vi "Manual Triggered Apodization 2.vi"() -> ()   [LabVIEW 2012]
uses:
  LabVIEW/user.lib/SpectralRadar.llb/Processing Parameter Int Selection.ctl
  LabVIEW/user.lib/SpectralRadar.llb/Calibration Selection.ctl
  LabVIEW/user.lib/SpectralRadar.llb/set Spectrum Output.vi
  LabVIEW/user.lib/SpectralRadar.llb/display Data 1D.vi
  LabVIEW/user.lib/SpectralRadar.llb/OCT Device.lvclass
  LabVIEW/user.lib/SpectralRadar.llb/Processing.lvclass
  LabVIEW/user.lib/SpectralRadar.llb/Raw Data.lvclass
  LabVIEW/user.lib/SpectralRadar.llb/Data.lvclass
panel:
  out "Waveform Graph":dbl[](graph)
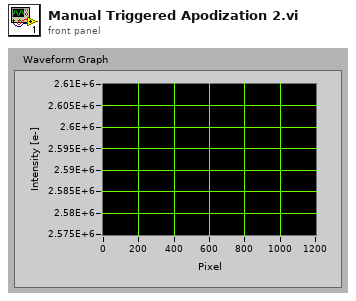
[diagram p1: front panel]
types:
  T1 = typedef "Processing.lvclass/Calibration Selection.ctl" = enum16{"Offset Errors", "Apodization Spectrum", "Apodization Vector", "Dispersion", "Chirp", "Extended Adjust", "Fixed Pattern"}
  T2 = typedef "Processing.lvclass/Processing Parameter Int Selection.ctl" = enum32{"Spectrum Averaging", "A-Scan Averaging", "B-Scan Averaging", "Zero Padding", "Number of Threads", "Fourier Averaging"}
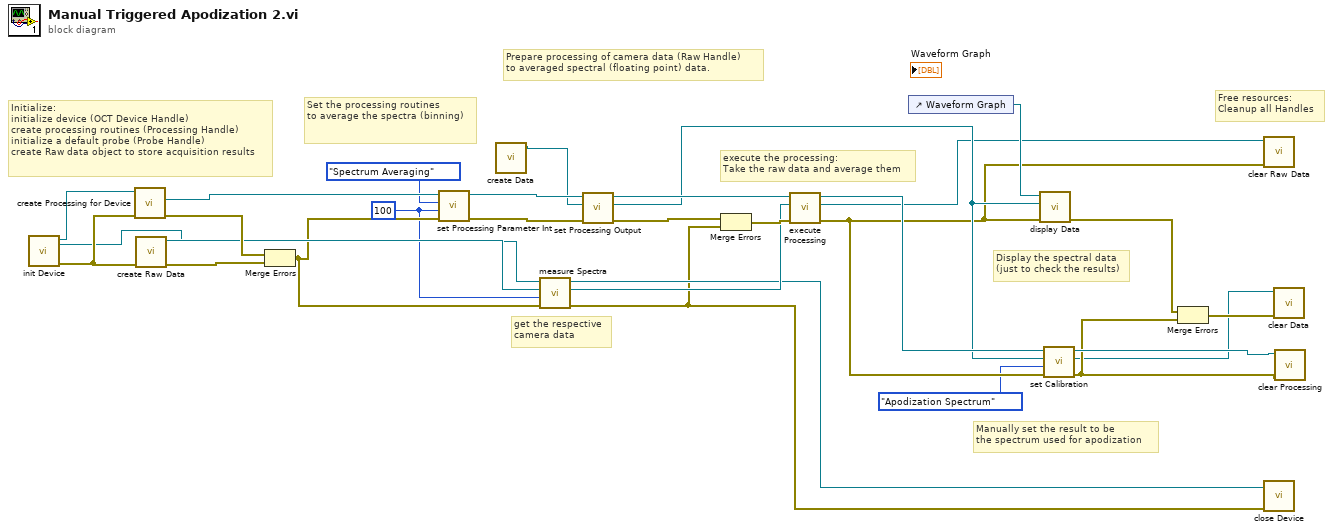
[diagram p0: block diagram]
diagram:
  w10 = 100 ("AScans")
  # "Free resources:\nCleanup all Handles"
  # "Manually set the result to be \nthe spectrum used for apodization"
  # "Display the spectral data\n(just to check the results)"
  # "execute the processing:\nTake the raw data and average them"
  # "get the respective \ncamera data"
  # "Prepare processing of camera data (Raw Handle)\nto averaged spectral (floating point) data."
  # "Set the processing routines \nto average the spectra (binning)"
  # "Initialize:\ninitialize device (OCT Device Handle)\ncreate processing routines (Processing Handle)\ninitialize a default probe (Probe Handle)\ncreate Raw data object to store acquisition results"
  n1 = call "init Device.vi"() -> ("error out"=w29:errorcluster, "OCTDevice"=w6:refnum<class "OCT Device.lvclass">)  [unwired: 6 in]
  n2 = call "create Processing for Device.vi"("error in (no error)"=w29, "OCTDevice"=w6) -> ("error out"=w27:errorcluster, "Processing"=w28:refnum<class "Processing.lvclass">)  [unwired: 3 in, 1 out]
  n3 = call "create Raw Data.vi"("error in (no error)"=w29) -> ("error out"=w26:errorcluster, "Raw Data"=w13:refnum<class "Raw Data.lvclass">)  [unwired: 5 in]
  n4 = Merge Errors(w27, w26) -> (w11:errorcluster)
  n5 = call "set Processing Parameter Int.vi"("error in (no error)"=w11, "Value"=w10, "Processing Paramter Int Selection"=Processing_Parameter_Int_Selection."Spectrum Averaging", "Processing in"=w28) -> ("error out"=w23:errorcluster, "Processing out"=w25:refnum<class "Processing.lvclass">)  [unwired: 2 in]
  n6 = call "create Data.vi"() -> ("Data"=w5:refnum<class "Data.lvclass">)  [unwired: 6 in, 1 out]
  n7 = call "measure Spectra.vi"("error in (no error)"=w11, "NumberOfSpectra"=w10, "Raw Data"=w13, "OCTDevice"=w6) -> ("error out"=w8:errorcluster, "Raw Data"=w12:refnum<class "Raw Data.lvclass">, "OCTDevice"=w9:refnum<class "OCT Device.lvclass">)  [unwired: 2 in]
  n8 = call-poly "set Processing Output.vi"("error in (no error)"=w23, "Data"=w5, "Processing"=w25) -> ("error out"=w15:errorcluster, "Data"=w19:refnum<class "Data.lvclass">, "Processing"=w22:refnum<class "Processing.lvclass">)  [unwired: 2 in]
  n9 = Merge Errors(w15, w8) -> (w14:errorcluster)
  n10 = call "execute Processing.vi"("error in (no error)"=w14, "Raw Data"=w12, "Processing"=w22) -> ("error out"=w16:errorcluster, "Raw Data"=w18:refnum<class "Raw Data.lvclass">, "Processing"=w20:refnum<class "Processing.lvclass">)  [unwired: 2 in]
  n11 = control-ref of="Waveform Graph"() -> (w21:refnum<vi>)
  n12 = call-poly "display Data.vi"("error in (no error)"=w16, "Data in"=w19, "WFGraph Refnum"=w21) -> ("error out"=w17:errorcluster)  [unwired: 2 in, 2 out]
  n13 = call "set Calibration.vi"("error in (no error)"=w16, "Calibration Data"=Calibration_Selection."Apodization Spectrum", "Data"=w19, "Processing"=w20) -> ("error out"=w3:errorcluster, "Data"=w1:refnum<class "Data.lvclass">, "Processing"=w4:refnum<class "Processing.lvclass">)  [unwired: 1 in]
  n14 = Merge Errors(w17, w3) -> (w2:errorcluster)
  n15 = call "clear Raw Data.vi"("error in (no error)"=w16, "Raw Data"=w18) -> ()  [unwired: 5 in, 1 out]
  n16 = call "close Device.vi"("error in (no error)"=w8, "OCTDevice"=w9) -> ()  [unwired: 5 in, 1 out]
  n17 = call "clear Data.vi"("error in (no error)"=w2, "Data"=w1) -> ()  [unwired: 5 in, 1 out]
  n18 = call "clear Processing.vi"("error in (no error)"=w3, "Processing"=w4) -> ()  [unwired: 5 in, 1 out]
